vi "Initialize Device.vi"(8 "error in (no error)":errorcluster, 9 "Reset (F)":bool, 10 "Resource Name":string, 11 "CS++DeviceActor in":refnum<class "CS++DeviceActor.lvclass">) -> (0 "error out":errorcluster, 3 "CS++DeviceActor out":refnum<class "CS++DeviceActor.lvclass">)   [LabVIEW 2013, in "CS++DeviceActor.lvlib" / "CS++DeviceActor.lvclass"]
doc: "Open connection to device and initialize."
uses:
  CS++DeviceActor.lvclass
  CS++DeviceActor.lvclass/CS++DeviceActor.ctl
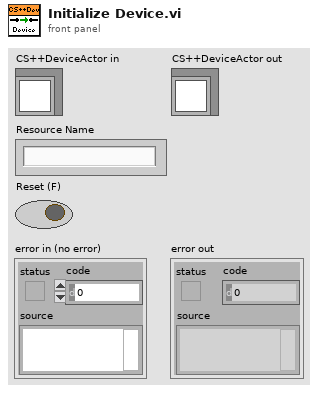
[diagram p1: front panel]
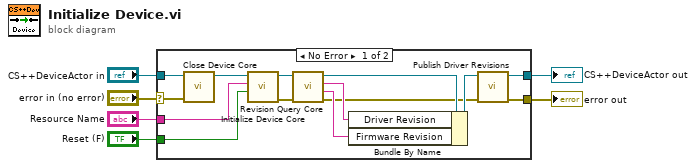
[diagram p0: block diagram]
diagram:
  n1 = case shown="No Error" "error in (no error)" {
    selector: "error in (no error)" -> [w16 w22]
    tunnel: [w7 w22] -> w5
    tunnel: [w9 w21] -> w3
    tunnel: "CS++DeviceActor in" -> [w18 w21]
    tunnel: "Resource Name" -> [w20 _]
    tunnel: "Reset (F)" -> [w19 _]
    frame No Error {
      n2 = call-dynamic "Close Device Core.vi"("error in (no error)"=w16, "CS++DeviceActor in"=w18) -> ("CS++DeviceActor out"=w17:refnum<class "CS++DeviceActor.lvclass">)  [unwired: 8 in, 1 out]
      n3 = call-dynamic "Initialize Device Core.vi"("Reset (F)"=w19, "Resource Name"=w20, "CS++DeviceActor in"=w17) -> ("error out"=w14:errorcluster, "CS++DeviceActor out"=w15:refnum<class "CS++DeviceActor.lvclass">)  [unwired: 7 in]
      n4 = call-dynamic "Revision Query Core.vi"("error in (no error)"=w14, "CS++DeviceActor in"=w15) -> ("error out"=w8:errorcluster, "Firmware Revision"=w11:string, "Driver Revision"=w12:string, "CS++DeviceActor out"=w13:refnum<class "CS++DeviceActor.lvclass">)  [unwired: 6 in]
      n5 = Bundle By Name(cluster=w13, "Driver Revision"=w12, "Firmware Revision"=w11) -> (w10:refnum<class "CS++DeviceActor.lvclass">)
      n6 = call "Publish Driver Revisions.vi"("error in (no error)"=w8, "CS++DeviceActor in"=w10) -> ("error out"=w7:errorcluster, "CS++DeviceActor out"=w9:refnum<class "CS++DeviceActor.lvclass">)  [unwired: 8 in]
    }
    frame Error {
    }
  }
  "error out" <- w5
  "CS++DeviceActor out" <- w3
